vi "CPTR Adjust Update.vi"(0 "Register Buses":T1[](array[typedef]), 5 "cptr adjust distances":u16[](array[numeric]), 11 "error in":errorcluster, 12 "sync.cptr.period":u16=1) -> (4 "Register Buses (out)":T1[](array[typedef]), 15 "error out":errorcluster)   [LabVIEW 2014, in "ni579x Synchronization v2 Host.lvlib"]
doc: "Based on the input measurements, calculate and set the CPTR Adjust values on all the devices."
uses:
  <instrlib>/ni579x/Synchronization/v2/Host/ni579x Synchronization v2 Host.lvlib
  <instrlib>/_niInstr/Register Bus/v0/Host/Public/Register Bus Session.ctl
  <instrlib>/_niInstr/Register Bus/v0/Host/Private/Session Data.ctl
  <instrlib>/ni579x/Synchronization/v2/Shared/ni579x Synchronization Register Addresses.ctl
  <instrlib>/ni579x/Config/v2/Shared/Types/ni579x Register Bus Subsystem ID.ctl
  <instrlib>/_niInstr/Register Bus/v0/Host/Public/Register Read Request.ctl
  <instrlib>/_niInstr/Register Bus/v0/Host/Public/Register Write.ctl
  <instrlib>/ni579x/Config/v2/Shared/ni579x Config v2 Shared.lvlib
  <instrlib>/_niInstr/Register Bus/v0/Host/niInstr Register Bus v0 Host.lvlib
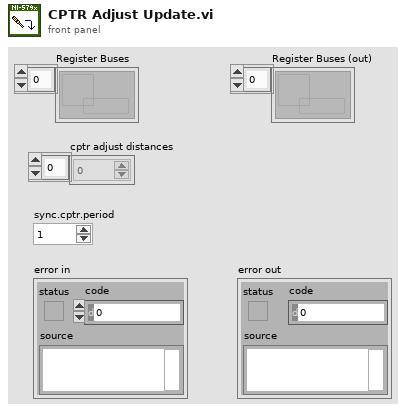
[diagram p1: front panel]
types:
  T1 = typedef "niInstr Register Bus v0 Host.lvlib/Register Bus Session.ctl" = refnum<queue>
  T2 = typedef "niInstr Register Bus v0 Host.lvlib/Register Read Request.ctl" = cluster{"subsystem":u8, "address":u16}
  T3 = typedef "ni579x Config v2 Shared.lvlib/ni579x Register Bus Subsystem ID.ctl" = u8
  T4 = typedef "ni579x Synchronization Register Addresses.ctl" = enum16{"Signature", "Current Version", "Oldest Compatible Version", "Scratch Register", "sync.master", "sync.meas.enable", "sync.meas.ready", "sync.meas.arm", "sync.meas.valid", "sync.meas.value", "sync.cptr.adjust", "sync.cptr.period", "sync.meas.oversample factor"}
  T5 = typedef "niInstr Register Bus v0 Host.lvlib/Register Write.ctl" = cluster{"subsystem":u8, "address":u16, "data":u32}
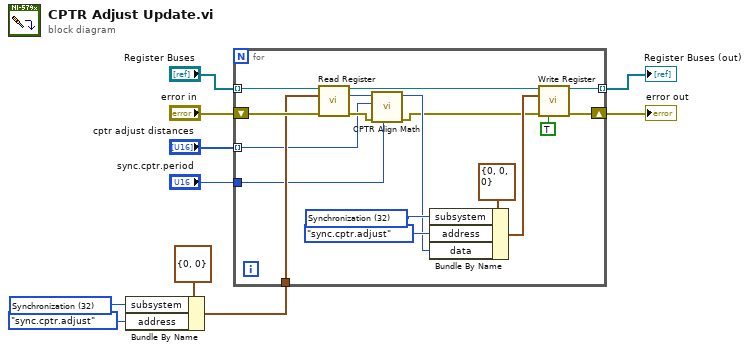
[diagram p0: block diagram]
diagram:
  w10 = T3 32 items=["FAM Register Operation"=0, "User Command"=16, "Synchronization"=32] ("Subsystem ID")
  n1 = Bundle By Name(cluster=T2 {"subsystem"=0, "address"=0} ("register read request"), "subsystem"=w10, "address"=ni579x_Synchronization_Register_Addresses."sync.cptr.adjust" ("Synchronization Registers")) -> (w7:T2)
  n2 = for {
    tunnel: [w17] -> w3 mode=indexing
    tunnel: "Register Buses" -> [w16] mode=indexing
    shift-right: [w18] -> w2
    shift-left: "error in" -> [w15]
    tunnel: w7 -> [w14]
    tunnel: "cptr adjust distances" -> [w12] mode=indexing
    tunnel: "sync.cptr.period" -> [w13]
    w26 = T3 32 items=["FAM Register Operation"=0, "User Command"=16, "Synchronization"=32] ("Subsystem ID")
    n3 = call <instrlib>:"Read Register.vi"("session in"=w16, "register read request"=w14, "error in"=w15) -> ("session out"=w20:T1, "data"=w23:u32, "error out"=w21:errorcluster)  [unwired: 10 in]
    n4 = call <instrlib>:"CPTR Align Math.vi"("sync.cptr.period"=w13, "error in"=w21, "measured cptr adjust distance"=w12, "sync.cptr.adjust"=w23) -> ("error out"=w19:errorcluster, "new cptr adjust"=w22:u16)  [unwired: 6 in]
    n5 = Bundle By Name(cluster=T5 {"subsystem"=0, "address"=0, "data"=0} ("register write"), "subsystem"=w26, "address"=ni579x_Synchronization_Register_Addresses."sync.cptr.adjust" ("Synchronization Registers"), "data"=w22) -> (w24:T5)
    n6 = call <instrlib>:"Write Register.vi"("session in"=w20, "register write"=w24, "error in"=w19, "wait until committed"=TRUE) -> ("session out"=w17:T1, "error out"=w18:errorcluster)  [unwired: 10 in]
  }
  "error out" <- w2
  "Register Buses (out)" <- w3
